vi "Configure Receive Parameters.vi"(7 "Micropulse # In":i32, 8 "error in (no error)":errorcluster, 9 "Receive Parameters":T1 {"Delay" format="%#_g us"; "Display Gate"."Length" min=0.0 max=64000.0 step=1.0 format="%#_g us"; "Display Gate"."Start" min=0.0 max=64000.0 step=1.0 format="%#_g us"; "Analogue Filtering"."Smoothing" min=1 max=11 step=1; "Gain" min=-6.0 max=70.0 step=0.25 format="%.2fdB"}, 11 "Test No.":u32) -> (0 "error out":errorcluster, 3 "Test No. out":u32, 5 "Micropulse # Out":i32)   [LabVIEW 2026, in "MicroPulse_Driver.lvlib"]
uses:
  MicroPulse_Driver.lvlib
  <instrlib>/MicroPulse/Public/Data/Datatypes/MP - receive parameters.ctl
  Data/Datatypes/MP - display gate.ctl
  <instrlib>/MicroPulse/Public/Data/Datatypes/MP - waveform type.ctl
  <instrlib>/MicroPulse/Public/Data/Datatypes/MP - analogue filter.ctl
  <instrlib>/MicroPulse/Public/Data/Datatypes/MP - frequency filter.ctl
  <instrlib>/MicroPulse/Public/Data/Datatypes/MP - digital filtering.ctl
  <instrlib>/MicroPulse/Public/Data/Datatypes/MP - high pass filter.ctl
  <instrlib>/MicroPulse/Public/Data/Datatypes/MP - low pass filter.ctl
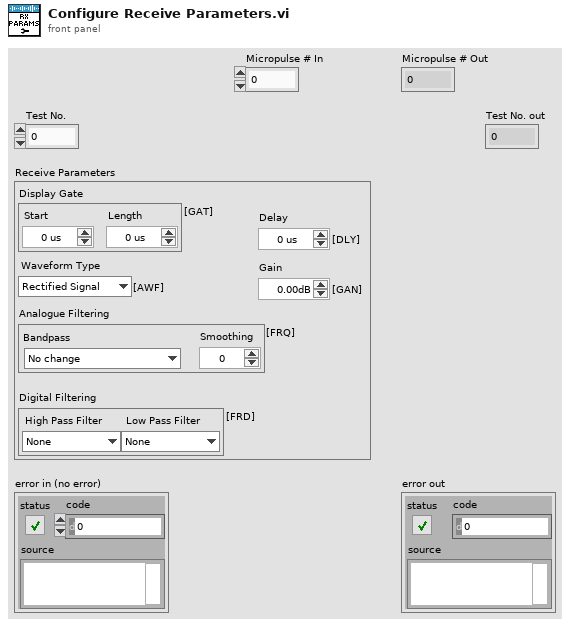
[diagram p1: front panel]
types:
  T1 = typedef "MicroPulse_Driver.lvlib/MP - receive parameters.ctl" = cluster{"Display Gate":T2, "Delay":dbl, "Waveform Type":T3, "Gain":dbl, "Analogue Filtering":T4, "Digital Filtering":T6}
  T2 = typedef "MicroPulse_Driver.lvlib/MP - display gate.ctl" = cluster{"Start":dbl, "Length":dbl}
  T3 = typedef "MicroPulse_Driver.lvlib/MP - waveform type.ctl" = enum16{"Rectified Signal", "RF Signal", "+Half Wave", "-Half Wave"}
  T4 = typedef "MicroPulse_Driver.lvlib/MP - analogue filter.ctl" = cluster{"Bandpass":T5, "Smoothing":u16}
  T5 = typedef "MicroPulse_Driver.lvlib/MP - frequency filter.ctl" = enum16{"No change", "1MHz Bandpass", "2MHz Bandpass", "4MHz Bandpass", "5MHz Bandpass", "10MHz Bandpass", "2.5-18MHz Broadband", "0.75-12MHz  Broadband", "0.5MHz Bandpass", "5MHz 2nd Order TOFD", "10MHz 2nd Order TOFD", "3.0-25MHz Broadband", "3.0-30MHz Broadband"}
  T6 = typedef "MicroPulse_Driver.lvlib/MP - digital filtering.ctl" = cluster{"High Pass Filter":T7, "Low Pass Filter":T8}
  T7 = typedef "MicroPulse_Driver.lvlib/MP - high pass filter.ctl" = enum16{"None", "0.7MHz", "1.5MHz", "4.0MHz", "7.5MHz", "10.0MHz", "User Defined"}
  T8 = typedef "MicroPulse_Driver.lvlib/MP - low pass filter.ctl" = enum16{"None", "1.8MHz", "3.0MHz", "6.0MHz", "8.0MHz", "12.0MHz", "User Defined"}
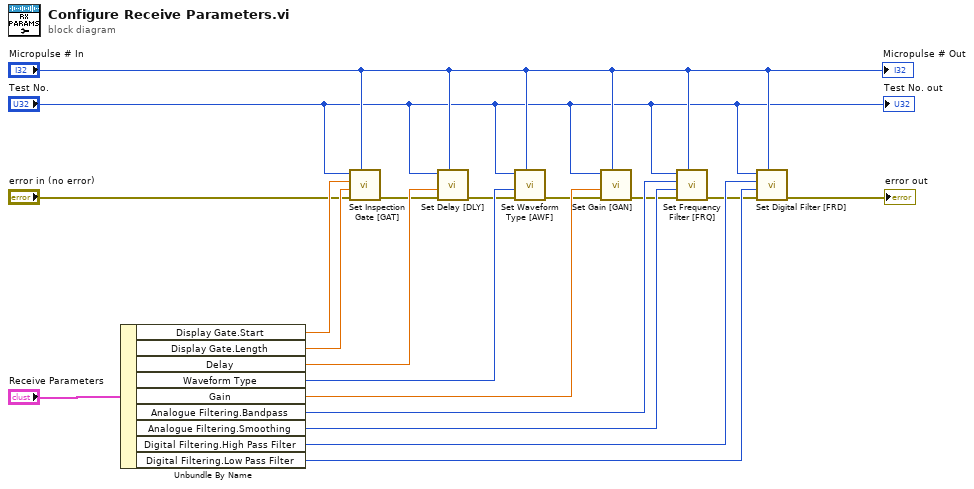
[diagram p0: block diagram]
diagram:
  n1 = Unbundle By Name("Receive Parameters") -> ("Display Gate.Start"=w11:dbl, "Display Gate.Length"=w12:dbl, "Delay"=w13:dbl, "Waveform Type"=w14:T3, "Gain"=w15:dbl, "Analogue Filtering.Bandpass"=w16:T5, "Analogue Filtering.Smoothing"=w17:u16, "Digital Filtering.High Pass Filter"=w18:T7, "Digital Filtering.Low Pass Filter"=w19:T8)
  n2 = call "Set Inspection Gate [GAT].vi"("Micropulse # In"="Micropulse # In", "error in (no error)"="error in (no error)", "Gate Length (us)"=w12, "Gate Start (us)"=w11, "Test Number"="Test No.") -> ("error out"=w5:errorcluster)  [unwired: 5 in, 1 out]
  n3 = call "Set Delay [DLY].vi"("Micropulse # In"="Micropulse # In", "error in (no error)"=w5, "Delay (us)"=w13, "Test Number"="Test No.") -> ("error out"=w6:errorcluster)  [unwired: 6 in, 1 out]
  n4 = call "Set Waveform Type [AWF].vi"("Micropulse # In"="Micropulse # In", "error in (no error)"=w6, "Waveform Type"=w14, "Test Number"="Test No.") -> ("error out"=w7:errorcluster)  [unwired: 6 in, 1 out]
  n5 = call "Set Gain [GAN].vi"("Micropulse # In"="Micropulse # In", "error in (no error)"=w7, "Gain (dB)"=w15, "Test Number"="Test No.") -> ("error out"=w8:errorcluster)  [unwired: 6 in, 1 out]
  n6 = call "Set Frequency Filter [FRQ].vi"("Micropulse # In"="Micropulse # In", "error in (no error)"=w8, "Smoothing"=w17, "Filter"=w16, "Test Number"="Test No.") -> ("error out"=w9:errorcluster)  [unwired: 5 in, 1 out]
  n7 = call "Set Digital Filter [FRD].vi"("Micropulse # In"="Micropulse # In", "error in (no error)"=w9, "Low Pass Filter"=w19, "High Pass Filter"=w18, "Test Number"="Test No.") -> ("error out"=→"error out":errorcluster)  [unwired: 5 in, 1 out]
  "Micropulse # Out" <- "Micropulse # In"
  "Test No. out" <- "Test No."
